vi "tcs_logEvent_SummaryState.vi"(8 "error in (no error)":errorcluster, 11 "logevent_SummaryState_Ctl":T1) -> (0 "error out":errorcluster, 2 "function return":i32, 3 "logevent_SummaryState_Ctl out":T1)   [LabVIEW 2016, in "SALLV_tcs.lvlib"]
doc: "int tcs_shm_logEvent_SummaryStateLV(tcs_logevent_SummaryStateLV *logevent_SummaryState_Ctl );"
uses:
  SALLV_tcs.lvlib
  DataTypes/logevent_SummaryState.ctl
  SALLV_tcs.so
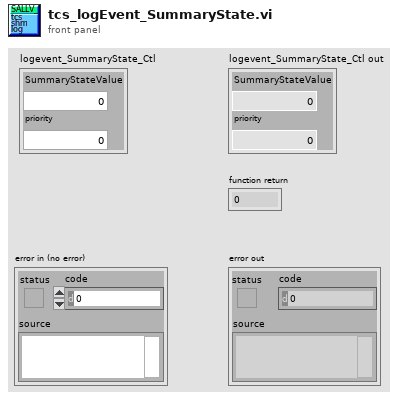
[diagram p1: front panel]
types:
  T1 = typedef "SALLV_tcs.lvlib/logevent_SummaryState.ctl" = cluster{"SummaryStateValue":i32, "priority":i32}
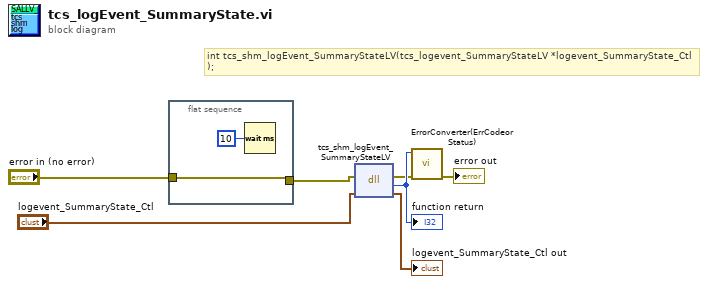
[diagram p0: block diagram]
diagram:
  # "int tcs_shm_logEvent_SummaryStateLV(tcs_logevent_SummaryStateLV *logevent_SummaryState_Ctl );"
  n1 = flat-sequence {
    tunnel: [w9] -> w1
    tunnel: "error in (no error)" -> [w9]
    frame #0 {
      n2 = Wait (ms)(milliseconds to wait=u32 10) -> ()  [unwired: 1 out]
    }
  }
  n3 = dll-call lib="home/andres/ct_tcs/ts_sallv_tcs/SALLV_tcs.*" fn="tcs_shm_logEvent_SummaryStateLV"(error in=w1, "logevent_SummaryState_Ctl"="logevent_SummaryState_Ctl") -> (error out=w4:errorcluster, w7:i32, "logevent_SummaryState_Ctl"=→"logevent_SummaryState_Ctl out":T1)  [unwired: 2 in, 1 out]
  "function return" <- w7
  n4 = call "ErrorConverter(ErrCodeorStatus).vi"("error in (no error)"=w4, "error code"=w7) -> ("error out"=→"error out":errorcluster)  [unwired: 9 in]
